vi "filt_gornoprzepustowy.vi"() -> ()   [LabVIEW 2012]
panel:
  out "Imie i nazwisko:":string
  out "Nr ćwiczenia:":string
  out "Data:":string
  in  "C":dbl
  in  "R":dbl
  out "Charakterystyka przesunięcia fazowego:":cluster{"X":dbl, "Y":dbl}[](graph)
  out "Charakterystyka wzmocnienia:":cluster{"X":dbl, "Y":dbl}[](graph)
  # "Program pokazuje charakterystykę wzmocnienia i przesunięcia fazowego filtra górnoprzepustowego \ndla podanych przez użytkownika wartości R (rezystancji) i C (pojemności elektrycznej)"
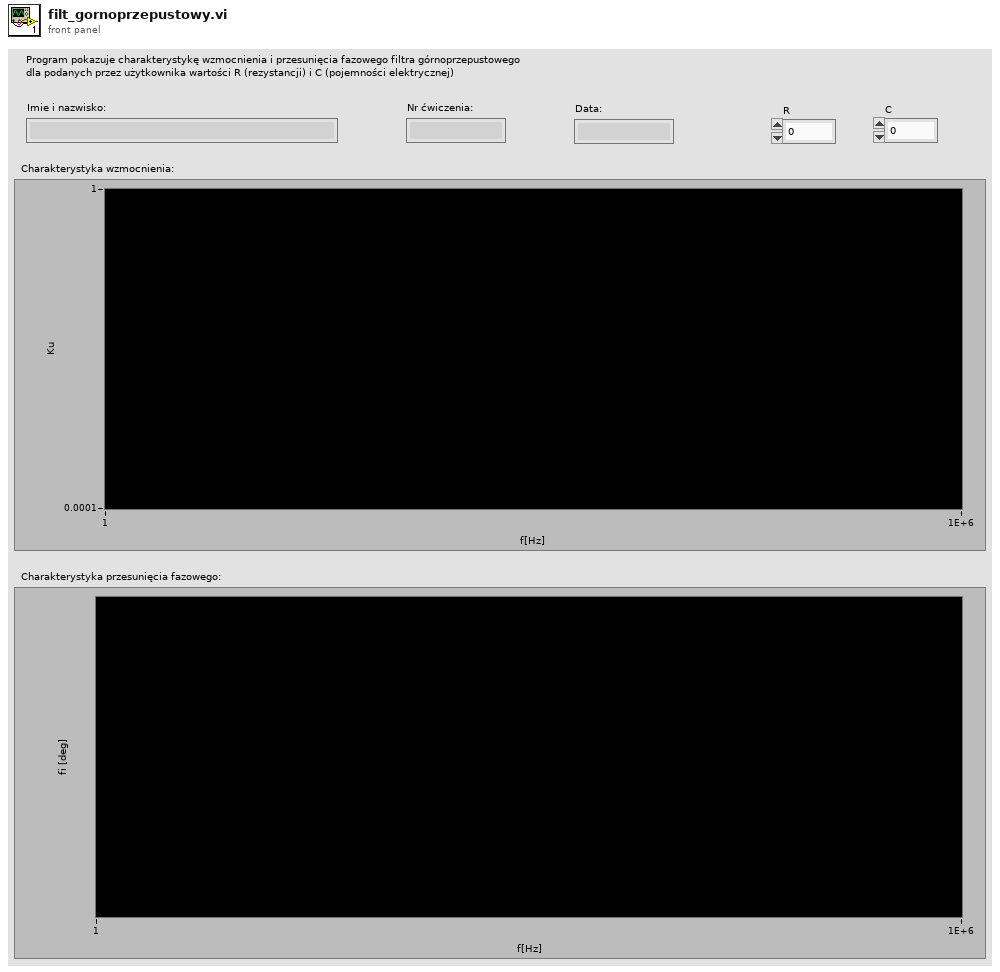
[diagram p1: front panel]
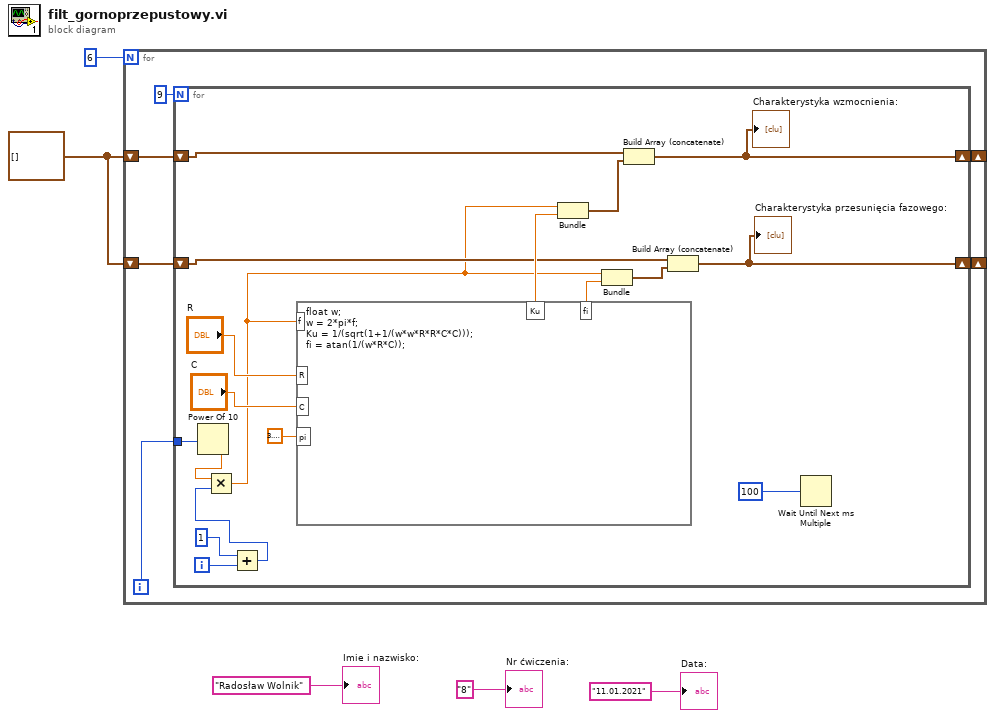
[diagram p0: block diagram]
diagram:
  w4 = cluster{"f":dbl, "Ku":dbl}[] []
  n1 = for {
    N: 6 -> [_]
    shift-right: [w9] -> _
    shift-left: w4 -> [w7]
    shift-right: [w8] -> _
    shift-left: w4 -> [w6]
    i -> [w10]
    n2 = for {
      N: 9 -> [_]
      shift-right: [w16] -> w9
      shift-left: w7 -> [w20]
      shift-right: [w15] -> w8
      shift-left: w6 -> [w18]
      tunnel: w10 -> [w24]
      i -> [w26]
      n3 = Power Of 10(x=w24) -> (10^x=w23:dbl)
      n4 = Add(x=1, y=w26) -> (x+y=w25:i32)
      n5 = Multiply(x=w23, y=w25) -> (x*y=w12:dbl)
      n6 = formula code="float w;\nw = 2*pi*f;\nKu = 1/(sqrt(1+1/(w*w*R*R*C*C)));\nfi = atan(1/(w*R*C));"("f"=w12, "R"="R", "C"="C", "pi"=3.141592653589793) -> ("Ku"=w22:dbl, "fi"=w21:dbl)
      n7 = Bundle(w12, "Ku"=w22) -> (w17:cluster{dbl, "Ku":dbl})  [unwired: 1 in]
      n8 = Bundle(w12, "fi"=w21) -> (w19:cluster{dbl, "fi":dbl})  [unwired: 1 in]
      n9 = Build Array (concatenate)(w18, w17) -> (w15:cluster{"f":dbl, "Ku":dbl}[])
      "Charakterystyka wzmocnienia:" <- w15
      n10 = Build Array (concatenate)(w20, w19) -> (w16:cluster{"f":dbl, "fi":dbl}[])
      "Charakterystyka przesunięcia fazowego:" <- w16
      n11 = Wait Until Next ms Multiple(millisecond multiple=100) -> ()  [unwired: 1 out]
    }
  }
  "Imie i nazwisko:" <- "Radosław Wolnik"
  "Data:" <- "11.01.2021"
  "Nr ćwiczenia:" <- "8"
